vi "Main.vi"() -> ()   [LabVIEW 2022 SP3]
doc: "This Continuous Measurement sample project is based on the Queued Message Handler template.\n\nThe Event Handling Loop generates messages based on user interface actions.\n\nThe Message Handling Loop processes messages generated by the Event Handling Loop, or by other messages. There are also Acquisition and Logging message handling loop subVIs, and a chart updating loop."
uses:
  Settings/Settings.ctl
  Acquisition/Network Configuration.ctl
  Logging/Logging Configuration.ctl
  controls/UI Data.ctl
  controls/UI State.ctl
  Acquisition/Network JSON.ctl
  support/Message Queue/Enqueue Message (Single).vi
  support/Message Queue/Enqueue Message (Array).vi
  <vilib>/Utility/error.llb/Error Cluster From Error Code.vi
  <vilib>/ErrorRing/Error Ring.xnode
  Acquisition/Acquisition.lvlib
  Logging/Logging.lvlib
  Settings/Settings.lvlib
  support/User Event - Stop/User Event - Stop.lvlib
  support/Message Queue/Message Queue.lvlib
  Settings/Settings Dialog.vi
panel:
  in  "Ignite":bool
  in  "Clear Console":bool
  in  "Deactuate 5":bool
  in  "Deactuate 4":bool
  in  "Deactuate 3":bool
  in  "Deactuate 2":bool
  in  "Deactuate 1":bool
  in  "Actuate 5":bool
  in  "Actuate 4":bool
  in  "Actuate 3":bool
  in  "Actuate 2":bool
  out "Pressure Transducers":waveform(dbl)[](graph)
  out "sensors":dbl[](array[numeric])
  out "Ignition State":bool
  out "Switch 5":bool
  out "Switch 4":bool
  out "Switch 3":bool
  out "Switch 2":bool
  out "Switch 1":bool
  out "Temperature":waveform(dbl)[](graph)
  out "Load Cells & Strain Gauges":waveform(dbl)[](graph)
  out "Console":string
  in  "Actuate 1":bool
  in  "Settings":bool
  in  "Restart Remote":bool
  in  "Connect":bool
  in  "Exit":bool
  # "LC 0"
  # "LC 1"
  # "LC 2"
  # "LC 3"
  # "SG 0"
  # "SG 1"
  # "TC 0"
  # "TC 1"
  # "TC 2"
  # "TC 3"
  # "PT 0"
  # "PT 1"
  # "PT 2"
  # "PT 3"
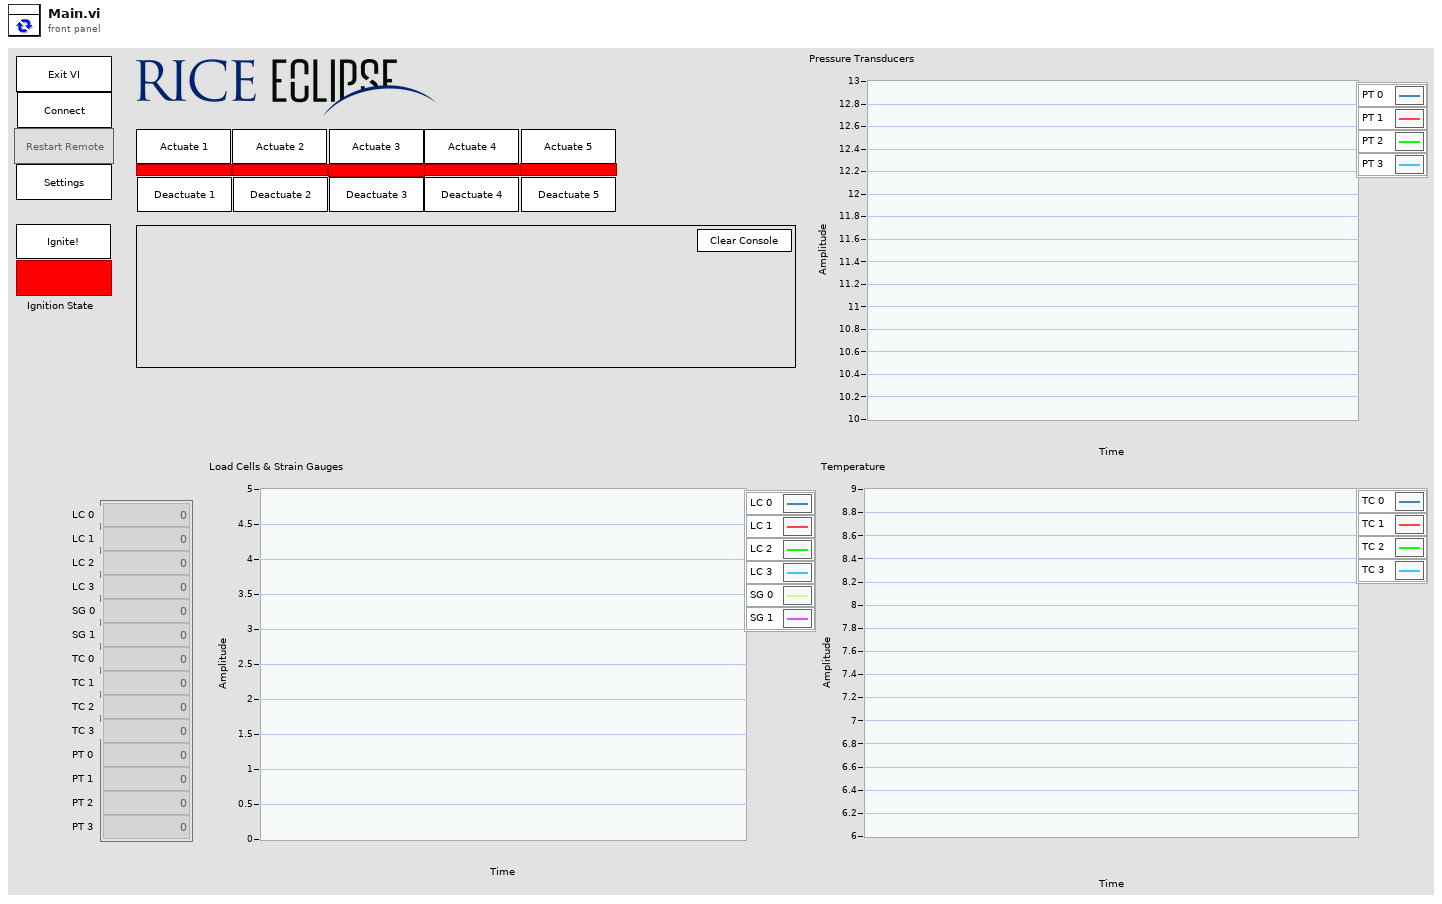
[diagram p1: front panel]
types:
  T1 = typedef "Network JSON.ctl" = cluster{"states":i32[], "timestamp":string, "console":string, "sensors":dbl[]}
  T2 = typedef "UI State.ctl" = enum16{"Idle", "Acquiring and Logging", "Waiting for Exit", "Waiting for Exit (Acq Stopped)", "Waiting for Exit (Log Stopped)", "Waiting for Stop", "Waiting for Stop (Acq Stopped)", "Waiting for Stop (Log Stopped)"}
  T3 = typedef "UI Data.ctl" = cluster{"Start Ref":refnum<vi>, "Stop Ref":refnum<vi>, "Settings Ref":refnum<vi>, "Exit Ref":refnum<vi>, "Console Ref":refnum<vi>, "Data Ref":refnum<vi>}
  T4 = typedef "Settings.lvlib/Settings.ctl" = cluster{"Network Configuration":T5, "Logging Configuration":T6}
  T5 = typedef "Acquisition.lvlib/Network Configuration.ctl" = cluster{"IP Address":string, "Port":dbl, "TCP Network Connection Refnum":refnum<k5>}
  T6 = typedef "Logging.lvlib/Logging Configuration.ctl" = cluster{"Log File Base Path":path, "TDMS File Reference":refnum<k34>}
  T7 = typedef "Message Queue.lvlib/All Message Queues.ctl" = cluster{"UI":refnum<queue>, "Acquisition":refnum<queue>, "Logging":refnum<queue>, "Sending":refnum<queue>}
  T8 = cluster{"command":string, "driver":i32, "value":i32}
  T9 = cluster{"[0]":bool, "[1]":bool, "[2]":bool, "[3]":bool, "[4]":bool, "[5]":bool, "[6]":bool, "[7]":bool, "[8]":bool}
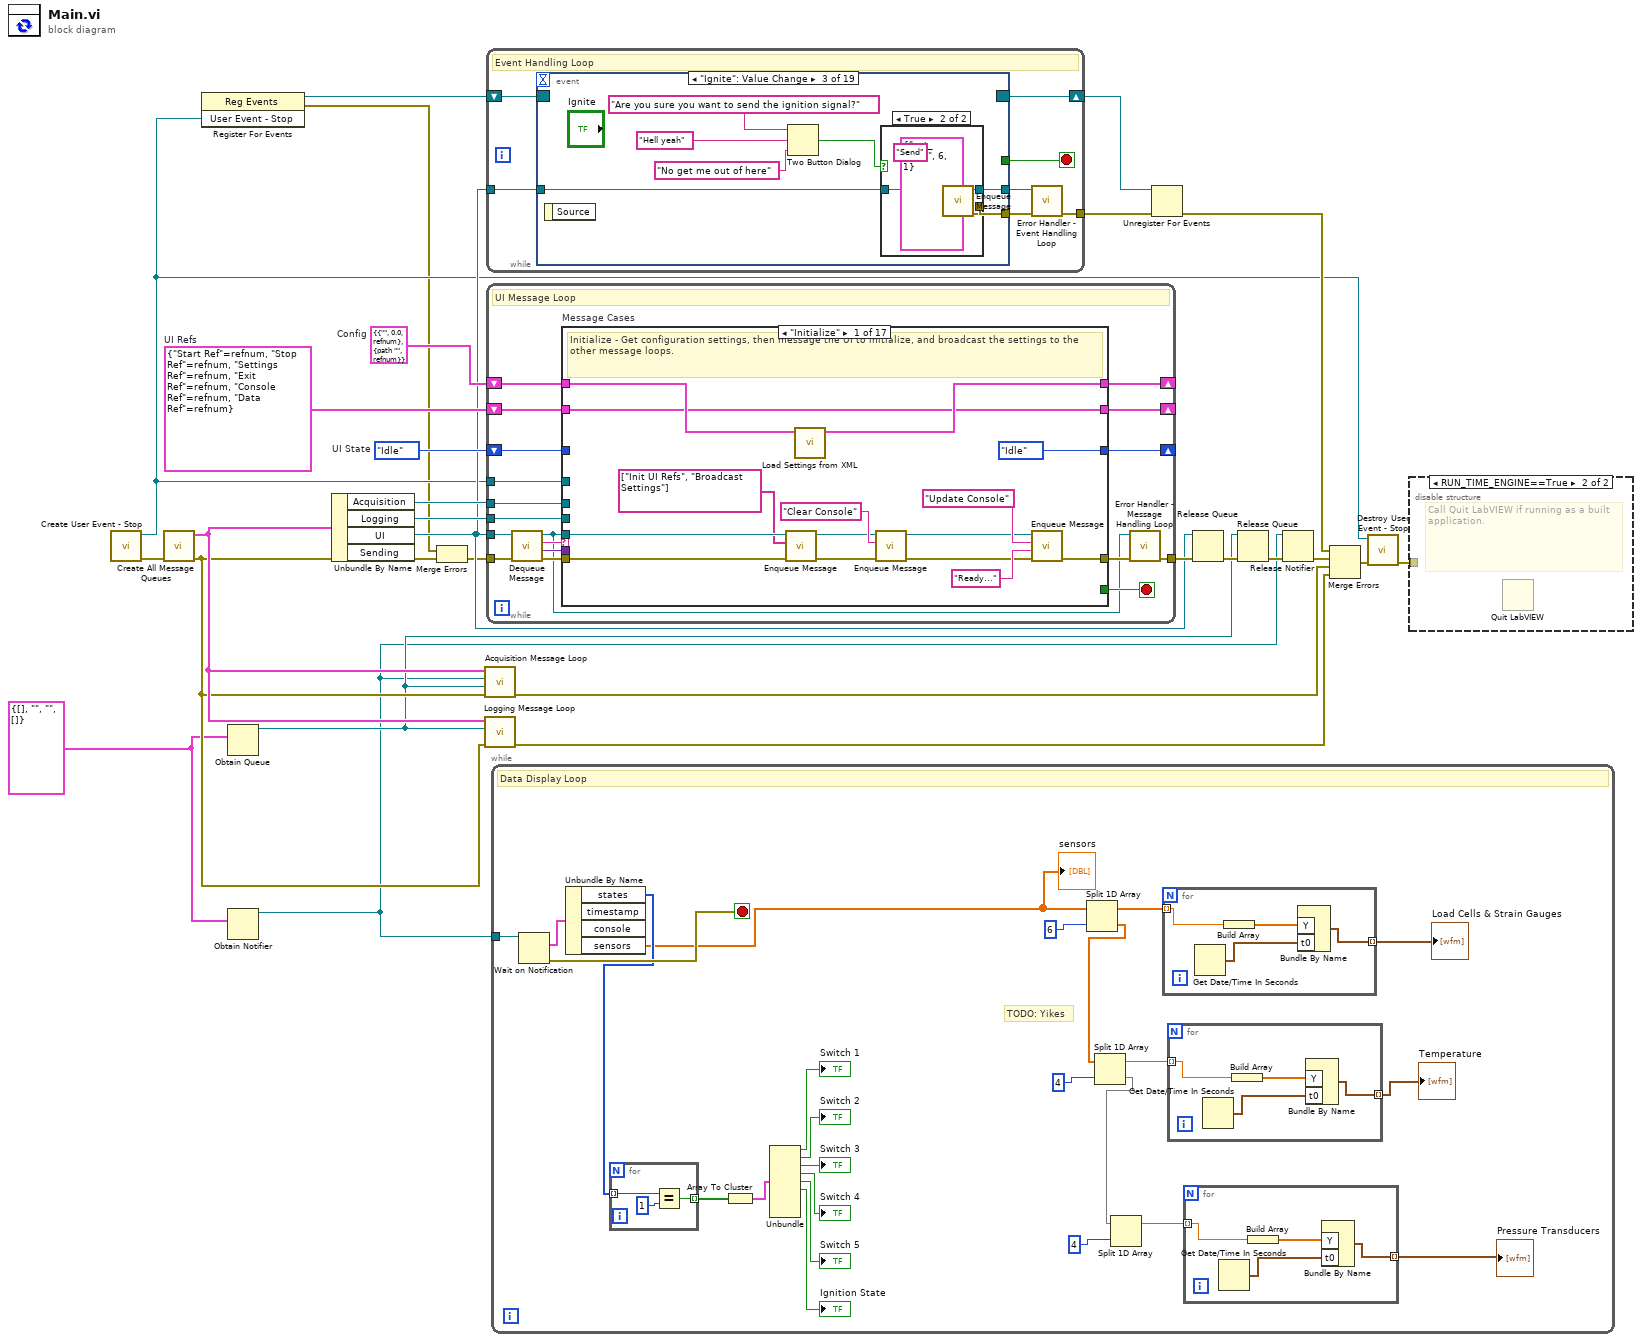
[diagram p0: block diagram]
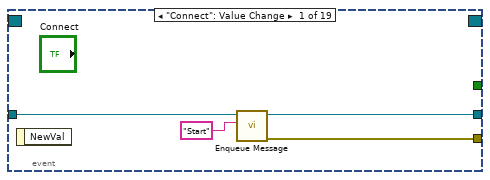
[diagram p3: hidden frame]
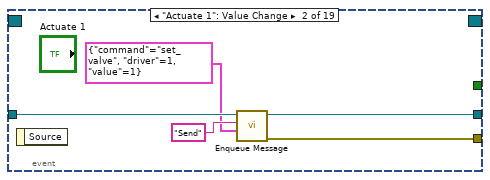
[diagram p4: hidden frame]
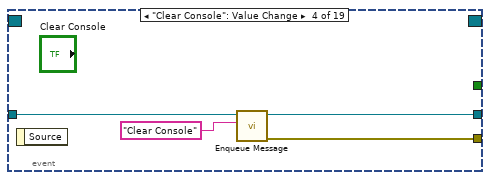
[diagram p6: hidden frame]
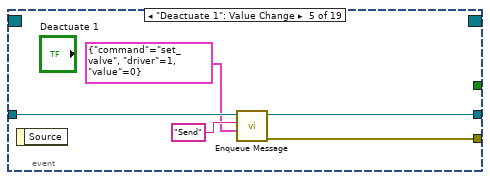
[diagram p7: hidden frame]
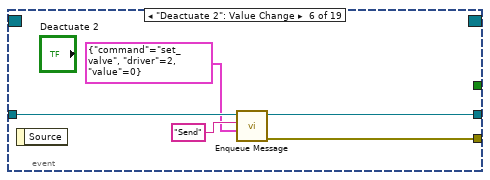
[diagram p8: hidden frame]
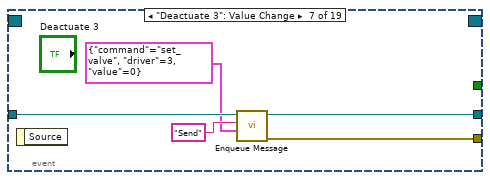
[diagram p9: hidden frame]
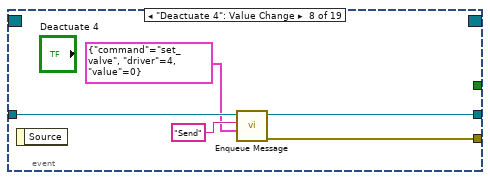
[diagram p10: hidden frame]
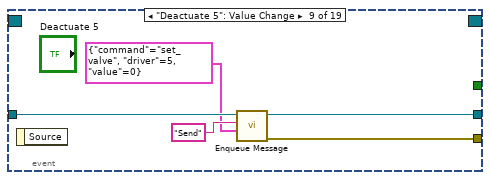
[diagram p11: hidden frame]
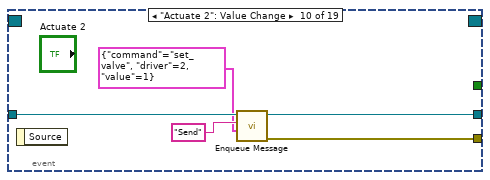
[diagram p12: hidden frame]
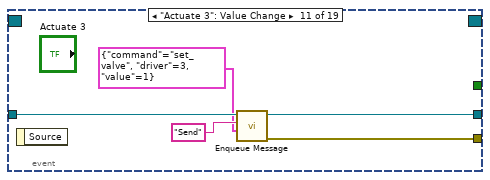
[diagram p13: hidden frame]
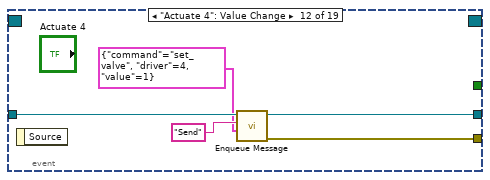
[diagram p14: hidden frame]
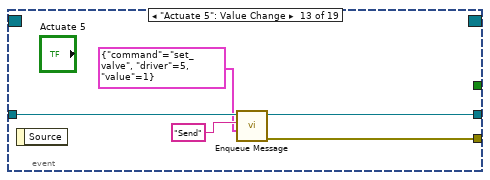
[diagram p15: hidden frame]
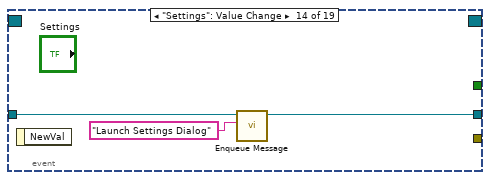
[diagram p16: hidden frame]
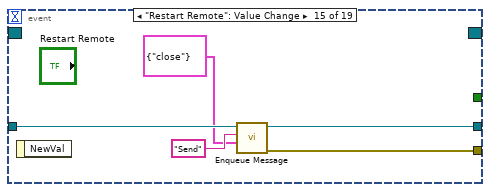
[diagram p17: hidden frame]
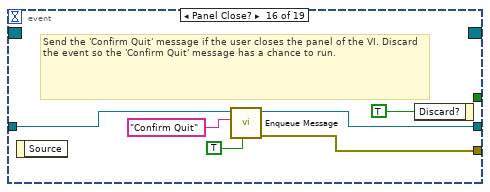
[diagram p18: hidden frame]
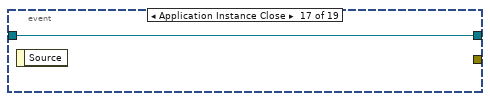
[diagram p19: hidden frame]
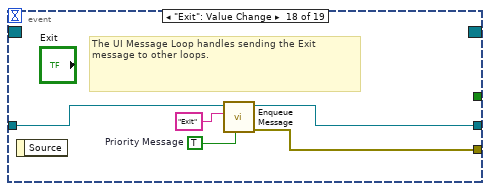
[diagram p20: hidden frame]
diagram:
  w2 = T1 {"states"=[], "timestamp"="", "console"="", "sensors"=[]} ("Network JSON")
  w14 = UI_State."Idle"  # UI State
  w17 = T3 {"Start Ref"=refnum, "Stop Ref"=refnum, "Settings Ref"=refnum, "Exit Ref"=refnum, "Console Ref"=refnum, "Data Ref"=refnum}  # UI Refs
  w20 = T4 {"Network Configuration"={"IP Address"="", "Port"=0.0, "TCP Network Connection Refnum"=refnum}, "Logging Configuration"={"Log File Base Path"=path "", "TDMS File Reference"=refnum}}  # Config
  n1 = call "Create User Event - Stop.vi"() -> ("error out"=w24:errorcluster, "User Event - Stop"=w5:refnum<user-event>)  [unwired: 10 in]
  n2 = call "Create All Message Queues.vi"("error in (no error)"=w24) -> ("error out"=w21:errorcluster, "Message Queues out"=w23:T7)  [unwired: 9 in]
  n3 = register-events(w5) -> (reference out=w6:refnum<event-registration>, error out=w3:errorcluster)  [unwired: 2 in]
  n4 = Obtain Queue(element data type=w2) -> (queue out=w7:refnum<queue>)  [unwired: 4 in, 2 out]
  n5 = Obtain Notifier(notification data type=w2) -> (notifier out=w1:refnum<notifier>)  [unwired: 3 in, 2 out]
  n6 = Unbundle By Name(w23) -> ("Acquisition"=w16:refnum<queue>, "Logging"=w15:refnum<queue>, "UI"=w12:refnum<queue>)  [unwired: 1 out]
  n7 = Merge Errors(w3, w21) -> (w4:errorcluster)
  n8 = call "Acquisition Message Loop.vi"("error in (no error)"=w21, "Data Queue"=w7, "Data Notifier"=w1, "Message Queues"=w23) -> ("error out"=w25:errorcluster)  [unwired: 7 in]
  n9 = call "Logging Message Loop.vi"("error in (no error)"=w21, "Data Queue"=w7, "Message Queues"=w23) -> ("error out"=w22:errorcluster)  [unwired: 8 in]
  n10 = while {
    tunnel: w12 -> [w33]
    tunnel: [w30] -> w26
    shift-right: [w32] -> w18
    shift-left: w6 -> [w34]
    stop <- w31 stop-if-true
    # "Event Handling Loop"
    n11 = event shown="[2] \"Ignite\": Value Change" {
      selector: w34 -> [_ _ _ _ _ _ _ _ _ _ _ _ _ _ _ _ _ _ _]
      dyn-events: [_ _ _ _ _ _ _ _ _ _ _ _ _ _ _ _ _ _ _] -> w32
      timeout: _ -> [_ _ _ _ _ _ _ _ _ _ _ _ _ _ _ _ _ _ _]
      tunnel: [_ _ _ _ _ _ _ _ _ _ _ _ _ _ _ _ _ _ TRUE ("Discard?")] -> w31
      tunnel: w33 -> [w38 w43 w50 w60 w65 w70 w75 w80 w85 w90 w95 w100 w105 w107 w112 w117 w120 w122 w126]
      tunnel: [w36 w41 w49 w58 w63 w68 w73 w78 w83 w88 w93 w98 w103 _ w111 w115 _ w125 _] -> w29
      tunnel: [w35 w40 w48 w57 w62 w67 w72 w77 w82 w87 w92 w97 w102 w106 w110 w116 w120 w121 w126] -> w28
      event "Connect": Value Change {
        n12 = event-data() -> ()  [unwired: 1 in, 1 out]
        n13 = call-poly "Enqueue Message.vi"("Message"="Start", "Message Queue"=w38) -> ("error out"=w36:errorcluster, "dup Message Queue"=w35:refnum<queue>)  [unwired: 8 in]
      }
      event "Actuate 1": Value Change {
        n14 = event-data() -> ()  [unwired: 1 in, 1 out]
        n15 = call-poly "Enqueue Message.vi"("Message Data"=T8 {"command"="set_valve", "driver"=1, "value"=1}, "Message"="Send", "Message Queue"=w43) -> ("error out"=w41:errorcluster, "dup Message Queue"=w40:refnum<queue>)  [unwired: 7 in]
      }
      event "Ignite": Value Change {
        n16 = event-data() -> ()  [unwired: 1 in, 1 out]
        n17 = Two Button Dialog(message="Are you sure you want to send the ignition signal?", 1:"No get me out of here", 2:"Hell yeah") -> (T button?=w44:bool)
        n18 = case shown="True" w44 {
          tunnel: w50 -> [w51 w56]
          tunnel: [_ w54] -> w49
          tunnel: [w51 w53] -> w48
          frame False {
          }
          frame True {
            n19 = call-poly "Enqueue Message.vi"("Message Data"=T8 {"command"="set_valve", "driver"=6, "value"=1}, "Message"="Send", "Message Queue"=w56) -> ("error out"=w54:errorcluster, "dup Message Queue"=w53:refnum<queue>)  [unwired: 7 in]
          }
        }
      }
      event "Clear Console": Value Change {
        n20 = event-data() -> ()  [unwired: 1 in, 1 out]
        n21 = call-poly "Enqueue Message.vi"("Message"="Clear Console", "Message Queue"=w60) -> ("error out"=w58:errorcluster, "dup Message Queue"=w57:refnum<queue>)  [unwired: 8 in]
      }
      event "Deactuate 1": Value Change {
        n22 = event-data() -> ()  [unwired: 1 in, 1 out]
        n23 = call-poly "Enqueue Message.vi"("Message Data"=T8 {"command"="set_valve", "driver"=1, "value"=0}, "Message"="Send", "Message Queue"=w65) -> ("error out"=w63:errorcluster, "dup Message Queue"=w62:refnum<queue>)  [unwired: 7 in]
      }
      event "Deactuate 2": Value Change {
        n24 = event-data() -> ()  [unwired: 1 in, 1 out]
        n25 = call-poly "Enqueue Message.vi"("Message Data"=T8 {"command"="set_valve", "driver"=2, "value"=0}, "Message"="Send", "Message Queue"=w70) -> ("error out"=w68:errorcluster, "dup Message Queue"=w67:refnum<queue>)  [unwired: 7 in]
      }
      event "Deactuate 3": Value Change {
        n26 = event-data() -> ()  [unwired: 1 in, 1 out]
        n27 = call-poly "Enqueue Message.vi"("Message Data"=T8 {"command"="set_valve", "driver"=3, "value"=0}, "Message"="Send", "Message Queue"=w75) -> ("error out"=w73:errorcluster, "dup Message Queue"=w72:refnum<queue>)  [unwired: 7 in]
      }
      event "Deactuate 4": Value Change {
        n28 = event-data() -> ()  [unwired: 1 in, 1 out]
        n29 = call-poly "Enqueue Message.vi"("Message Data"=T8 {"command"="set_valve", "driver"=4, "value"=0}, "Message"="Send", "Message Queue"=w80) -> ("error out"=w78:errorcluster, "dup Message Queue"=w77:refnum<queue>)  [unwired: 7 in]
      }
      event "Deactuate 5": Value Change {
        n30 = event-data() -> ()  [unwired: 1 in, 1 out]
        n31 = call-poly "Enqueue Message.vi"("Message Data"=T8 {"command"="set_valve", "driver"=5, "value"=0}, "Message"="Send", "Message Queue"=w85) -> ("error out"=w83:errorcluster, "dup Message Queue"=w82:refnum<queue>)  [unwired: 7 in]
      }
      event "Actuate 2": Value Change {
        n32 = event-data() -> ()  [unwired: 1 in, 1 out]
        n33 = call-poly "Enqueue Message.vi"("Message Data"=T8 {"command"="set_valve", "driver"=2, "value"=1}, "Message"="Send", "Message Queue"=w90) -> ("error out"=w88:errorcluster, "dup Message Queue"=w87:refnum<queue>)  [unwired: 7 in]
      }
      event "Actuate 3": Value Change {
        n34 = event-data() -> ()  [unwired: 1 in, 1 out]
        n35 = call-poly "Enqueue Message.vi"("Message Data"=T8 {"command"="set_valve", "driver"=3, "value"=1}, "Message"="Send", "Message Queue"=w95) -> ("error out"=w93:errorcluster, "dup Message Queue"=w92:refnum<queue>)  [unwired: 7 in]
      }
      event "Actuate 4": Value Change {
        n36 = event-data() -> ()  [unwired: 1 in, 1 out]
        n37 = call-poly "Enqueue Message.vi"("Message Data"=T8 {"command"="set_valve", "driver"=4, "value"=1}, "Message"="Send", "Message Queue"=w100) -> ("error out"=w98:errorcluster, "dup Message Queue"=w97:refnum<queue>)  [unwired: 7 in]
      }
      event "Actuate 5": Value Change {
        n38 = event-data() -> ()  [unwired: 1 in, 1 out]
        n39 = call-poly "Enqueue Message.vi"("Message Data"=T8 {"command"="set_valve", "driver"=5, "value"=1}, "Message"="Send", "Message Queue"=w105) -> ("error out"=w103:errorcluster, "dup Message Queue"=w102:refnum<queue>)  [unwired: 7 in]
      }
      event "Settings": Value Change {
        n40 = event-data() -> ()  [unwired: 1 in, 1 out]
        n41 = call-poly "Enqueue Message.vi"("Message"="Launch Settings Dialog", "Message Queue"=w107) -> ("dup Message Queue"=w106:refnum<queue>)  [unwired: 8 in, 1 out]
      }
      event "Restart Remote": Value Change {
        n42 = event-data() -> ()  [unwired: 1 in, 1 out]
        n43 = call-poly "Enqueue Message.vi"("Message Data"=cluster{"command":string} {"command"="close"}, "Message"="Send", "Message Queue"=w112) -> ("error out"=w111:errorcluster, "dup Message Queue"=w110:refnum<queue>)  [unwired: 7 in]
      }
      event Panel Close? {
        # "Send the 'Confirm Quit' message if the user closes the panel of the VI. Discard the event so the 'Confirm Quit' message has a chance to run."
        n44 = event-data() -> ()  [unwired: 1 in, 1 out]
        n45 = call-poly "Enqueue Message.vi"("Priority Message? (F)"=TRUE, "Message"="Confirm Quit", "Message Queue"=w117) -> ("error out"=w115:errorcluster, "dup Message Queue"=w116:refnum<queue>)  [unwired: 7 in]
        n46 = event-data("Discard?"=TRUE) -> ()  [unwired: 1 in, 1 out]
      }
      event Application Instance Close {
        n47 = event-data() -> ()  [unwired: 1 in, 1 out]
      }
      event "Exit": Value Change {
        w123 = TRUE  # Priority Message
        # "The UI Message Loop handles sending the Exit message to other loops."
        n48 = event-data() -> ()  [unwired: 1 in, 1 out]
        n49 = call-poly "Enqueue Message.vi"("Priority Message? (F)"=w123, "Message"="Exit", "Message Queue"=w122) -> ("error out"=w125:errorcluster, "dup Message Queue"=w121:refnum<queue>)  [unwired: 7 in]
      }
      event User Event {
        # "The Message Handling Loop processed an \"Exit\" message, which fired this event to stop the Event Handling Loop."
        n50 = event-data() -> ()  [unwired: 1 in, 1 out]
        n51 = local write "Console"("Exit" ("Exit String")) -> ()
      }
    }
    n52 = call "Error Handler - Event Handling Loop.vi"("error in (no error)"=w29, "Message Queue"=w28) -> ("dup error in"=w30:errorcluster)  [unwired: 8 in, 1 out]
  }
  n53 = while {
    tunnel: w12 -> [w140]
    tunnel: w5 -> [w145]
    shift-right: [w139] -> _
    shift-left: w20 -> [w138]
    shift-right: [w136] -> _
    shift-left: w17 -> [w137]
    tunnel: w16 -> [w135]
    tunnel: w15 -> [w134]
    shift-right: [w129] -> _
    shift-left: w14 -> [w130]
    tunnel: w4 -> [w144]
    tunnel: [w133] -> w27
    stop <- w146 stop-if-true
    # "UI Message Loop"
    n54 = call "Dequeue Message.vi"("error in (no error)"=w144, "Message Queue"=w140) -> ("error out"=w143:errorcluster, "Message Data"=w141:variant, "Message"=w142:string, "dup Message Queue"=w131:refnum<queue>)  [unwired: 6 in]
    n55 = case "Message Cases" shown="\"Initialize\"" w142 {
      selector: w142 -> [_ _ _ _ _ _ _ _ _ _ _ _ _ _ _ _ w410]
      tunnel: w131 -> [w155 _ _ w210 _ w235 w260 _ w300 w310 w328 _ _ _ _ w397 _]
      tunnel: w143 -> [w154 w175 w187 w209 w229 w236 w261 w288 w302 w312 w327 w356 w373 w380 w388 w403 _]
      tunnel: [w159 w175 w188 w192 w230 w233 w258 w294 w295 w315 w326 w366 w372 w379 w391 w408 w409] -> w132
      tunnel: [_ _ _ _ _ _ _ _ _ _ _ TRUE _ _ _ _ _] -> w146
      tunnel: w141 -> [_ _ w186 _ _ _ _ _ _ w316 _ w354 _ _ w386 w402 _]
      tunnel: w145 -> [_ _ _ _ _ _ _ _ _ _ _ w367 _ _ _ _ _]
      tunnel: [w160 w174 w183 w208 w228 w239 w264 w292 w299 w320 w331 w365 w371 w378 w382 w405 w413] -> w139
      tunnel: w138 -> [w161 w174 w183 w208 w228 w239 w264 w292 w303 w320 w331 w365 w371 w378 w383 w405 w413]
      tunnel: w137 -> [w156 w173 w182 w205 w227 w238 w263 w286 w297 w319 w330 w364 w370 w375 w390 w407 w412]
      tunnel: [w156 w171 w182 w205 w227 w238 w263 w286 w297 w319 w330 w364 w370 w375 w390 w407 w412] -> w136
      tunnel: w135 -> [_ _ _ w191 w214 _ _ w285 _ _ _ w363 _ _ _ _ _]
      tunnel: w134 -> [_ _ _ w194 w217 _ _ w284 _ _ _ w362 _ _ _ _ _]
      tunnel: w130 -> [_ _ w181 _ w211 w237 w262 w283 w296 w314 w329 _ w369 w377 w389 w406 w411]
      tunnel: [UI_State."Idle" ("UI State") UI_State."Idle" ("UI State") w181 UI_State."Acquiring and Logging" ("UI State") w212 w234 w259 w283 w296 w314 w325 UI_State."Idle" ("UI State") w369 w377 w389 w406 w411] -> w129
      frame "Initialize" {
        # "Initialize - Get configuration settings, then message the UI to initialize, and broadcast the settings to the other message loops."
        n56 = call-poly "Enqueue Message.vi"("error in (no error)"=w154, "Message Array"=string[] ["Init UI Refs", "Broadcast Settings"], "Message Queue"=w155) -> ("error out"=w151:errorcluster, "dup Message Queue"=w148:refnum<queue>)  [unwired: 7 in]
        n57 = call "Load Settings from XML.vi"("Settings in"=w161) -> ("Settings out"=w160:T4)  [unwired: 9 in, 1 out]
        n58 = call-poly "Enqueue Message.vi"("error in (no error)"=w151, "Message"="Clear Console", "Message Queue"=w148) -> ("error out"=w150:errorcluster, "dup Message Queue"=w147:refnum<queue>)  [unwired: 7 in]
        n59 = call-poly "Enqueue Message.vi"("error in (no error)"=w150, "Message Data"="Ready..." ("Ready..."), "Message"="Update Console", "Message Queue"=w147) -> ("error out"=w159:errorcluster)  [unwired: 6 in, 1 out]
      }
      frame "Init UI Refs" {
        # "Enable: Start, Exit, Settings\nDisable: Stop"
        # "Init UI Refs - Store control references for UI controls.  Also enable/disable controls appropriately."
        n60 = control-ref of="Connect"() -> (w165:refnum<vi>)
        n61 = control-ref of="Restart Remote"() -> (w166:refnum<vi>)
        n62 = control-ref of="Settings"() -> (w164:refnum<vi>)
        n63 = control-ref of="Exit"() -> (w163:refnum<vi>)
        n64 = control-ref of="Console"() -> (w172:refnum<vi>)
        n65 = Bundle By Name(cluster=w173, "Start Ref"=w165, "Stop Ref"=w166, "Settings Ref"=w164, "Exit Ref"=w163, "Console Ref"=w172) -> (w171:T3)
        n66 = Build Array(w165, w164, w163) -> (w169:refnum<vi>[])
        n67 = Build Array(w166) -> (w168:refnum<vi>[])
        n68 = call "Set Enable State on Multiple Controls.vi"("Enable?"=TRUE, "Controls"=w169) -> ()  [unwired: 10 in]
        n69 = call "Set Enable State on Multiple Controls.vi"("Enable?"=FALSE, "Controls"=w168) -> ()  [unwired: 10 in]
      }
      frame "Update Console" {
        # "Update Status - Convert the message data to a string to display in the Status indicator."
        n70 = property on="Console" class="Str"() -> ("Text.Text"=w179:string)  [unwired: 2 in, 2 out]
        n71 = Variant To Data(error in=w187, type="", Variant=w186) -> (data=w178:string, error out=w184:errorcluster)
        n72 = Concatenate Strings(w179, "\r\n", w178) -> (→"Console":string)
        n73 = property on="Console" class="Str"("Text.Scroll Position"=1000000) -> ()  [unwired: 2 in, 2 out]
        n74 = Merge Errors(w184) -> (w188:errorcluster)
      }
      frame "Start" {
        # "Message Acquisition and Logging loops to start."
        # "Enable: Stop\nDisable: Start, Exit, Settings"
        # "Start - Enable/Disable buttons appropriately for an acquisition that has started, and update status display."
        n75 = Unbundle By Name(w205) -> ("Stop Ref"=w200:refnum<vi>, "Start Ref"=w199:refnum<vi>, "Exit Ref"=w198:refnum<vi>, "Settings Ref"=w197:refnum<vi>)
        n76 = call-poly "Enqueue Message.vi"("error in (no error)"=w209, "Message Data"="Acquiring and Logging..." ("Acquiring and Logging..."), "Message"="Update Console", "Message Queue"=w210) -> ("error out"=w196:errorcluster)  [unwired: 6 in, 1 out]
        n77 = Build Array(w199, w198, w197) -> (w203:refnum<vi>[])
        n78 = Build Array(w200) -> (w202:refnum<vi>[])
        n79 = call "Set Enable State on Multiple Controls.vi"("Enable?"=TRUE, "Controls"=w202) -> ()  [unwired: 10 in]
        n80 = call "Set Enable State on Multiple Controls.vi"("Enable?"=FALSE, "Controls"=w203) -> ()  [unwired: 10 in]
        n81 = call-poly "Enqueue Message.vi"("error in (no error)"=w196, "Message"="Start", "Message Queue"=w194) -> ("error out"=w193:errorcluster)  [unwired: 7 in, 1 out]
        n82 = call-poly "Enqueue Message.vi"("error in (no error)"=w193, "Message"="Start", "Message Queue"=w191) -> ("error out"=w192:errorcluster)  [unwired: 7 in, 1 out]
      }
      frame "Stop" {
        # "Message Acquisition and Logging loops to stop"
        # "Enable: Start, Exit, Settings\nDisable: Stop"
        # "Stop - Enable/Disable buttons appropriately for an acquisition that has stopped, and update status display."
        n83 = Unbundle By Name(w227) -> ("Stop Ref"=w222:refnum<vi>, "Start Ref"=w221:refnum<vi>, "Exit Ref"=w220:refnum<vi>, "Settings Ref"=w219:refnum<vi>)
        n84 = Build Array(w221, w220, w219) -> (w225:refnum<vi>[])
        n85 = Build Array(w222) -> (w224:refnum<vi>[])
        n86 = call "Set Enable State on Multiple Controls.vi"("Enable?"=FALSE, "Controls"=w224) -> ()  [unwired: 10 in]
        n87 = call "Set Enable State on Multiple Controls.vi"("Enable?"=TRUE, "Controls"=w225) -> ()  [unwired: 10 in]
        n88 = call-poly "Enqueue Message.vi"("error in (no error)"=w229, "Message"="Stop", "Message Queue"=w217) -> ("error out"=w216:errorcluster)  [unwired: 7 in, 1 out]
        n89 = case shown="\"Waiting for Exit\"" w211 {
          selector: w211 -> [w231 _]
          tunnel: [w231 UI_State."Waiting for Stop" ("UI State")] -> w212
          frame "Waiting for Exit" {
          }
          frame Default {
          }
        }
        n90 = call-poly "Enqueue Message.vi"("error in (no error)"=w216, "Message"="Stop", "Message Queue"=w214) -> ("error out"=w215:errorcluster)  [unwired: 7 in, 1 out]
        n91 = Merge Errors(w215) -> (w230:errorcluster)
      }
      frame "Acquisition Stopped" {
        # "Logic for determining what action to take when the acquisition has stopped."
        n92 = case shown="\"Waiting for Exit (Log Stopped)\"" w237 {
          selector: w237 -> [w241 _ _ _ _]
          tunnel: w236 -> [w240 w243 w245 w251 w257]
          tunnel: w235 -> [_ _ _ w249 w254]
          tunnel: [w241 UI_State."Waiting for Exit (Acq Stopped)" ("UI State") UI_State."Waiting for Stop (Acq Stopped)" ("UI State") UI_State."Idle" ("UI State") UI_State."Idle" ("UI State")] -> w234
          tunnel: [w240 w243 w245 w250 w255] -> w233
          frame Default {
          }
          frame "Waiting for Exit", "Waiting for Exit (Acq Stopped)" {
          }
          frame "Waiting for Stop", "Waiting for Stop (Acq Stopped)" {
          }
          frame "Waiting for Exit (Log Stopped)" {
            # "If we are waiting to exit, and the logging has already stopped, then the \"Acquisition Stopped\" message indicates that it is time to exit."
            n93 = call-poly "Enqueue Message.vi"("Priority Message? (F)"=TRUE, "error in (no error)"=w251, "Message"="Exit", "Message Queue"=w249) -> ("error out"=w250:errorcluster)  [unwired: 6 in, 1 out]
          }
          frame "Waiting for Stop (Log Stopped)" {
            # "If we are waiting to stop, and the logging has already stopped, then the \"Acquisition Stopped\" message indicates that it is time to stop."
            n94 = call-poly "Enqueue Message.vi"("error in (no error)"=w257, "Message Data"="Ready..." ("Ready..."), "Message"="Update Status", "Message Queue"=w254) -> ("error out"=w255:errorcluster)  [unwired: 6 in, 1 out]
          }
        }
      }
      frame "Logging Stopped" {
        # "Logic for determining what action to take when the logging has stopped."
        n95 = case shown="\"Waiting for Stop (Acq Stopped)\"" w262 {
          selector: w262 -> [w266 _ _ _ _]
          tunnel: w261 -> [w265 w268 w270 w276 w279]
          tunnel: w260 -> [_ _ _ w274 w278]
          tunnel: [w266 UI_State."Waiting for Exit (Log Stopped)" ("UI State") UI_State."Waiting for Stop (Log Stopped)" ("UI State") UI_State."Idle" ("UI State") UI_State."Idle" ("UI State")] -> w259
          tunnel: [w265 w268 w270 w275 w277] -> w258
          frame Default {
          }
          frame "Waiting for Exit", "Waiting for Exit (Log Stopped)" {
          }
          frame "Waiting for Stop", "Waiting for Stop (Log Stopped)" {
          }
          frame "Waiting for Exit (Acq Stopped)" {
            # "If we are waiting to exit, and the acquisition has already stopped, then the \"Logging Stopped\" message indicates that it is time to exit."
            n96 = call-poly "Enqueue Message.vi"("Priority Message? (F)"=TRUE, "error in (no error)"=w276, "Message"="Exit", "Message Queue"=w274) -> ("error out"=w275:errorcluster)  [unwired: 6 in, 1 out]
          }
          frame "Waiting for Stop (Acq Stopped)" {
            # "If we are waiting to stop, and the acquisition has already stopped, then the \"Logging Stopped\" message indicates that it is time to stop."
            n97 = call-poly "Enqueue Message.vi"("error in (no error)"=w279, "Message Data"="Ready..." ("Ready..."), "Message"="Update Console", "Message Queue"=w278) -> ("error out"=w277:errorcluster)  [unwired: 6 in, 1 out]
          }
        }
      }
      frame "Broadcast settings" {
        w287 = "Update Settings" ("Message")
        # "Broadcast settings - Send the 'Update Settings' message to the Logging and Acquisition message loops."
        n98 = Unbundle By Name(w292) -> ("Network Configuration"=w291:T5, "Logging Configuration"=w290:T6)
        n99 = call-poly "Enqueue Message.vi"("Message Data"=w291, "Message"=w287, "Message Queue"=w285) -> ("error out"=w293:errorcluster)  [unwired: 7 in, 1 out]
        n100 = call-poly "Enqueue Message.vi"("error in (no error)"=w293, "Message Data"=w290, "Message"=w287, "Message Queue"=w284) -> ("error out"=w289:errorcluster)  [unwired: 6 in, 1 out]
        n101 = Merge Errors(w289, w288) -> (w294:errorcluster)
      }
      frame "Launch Settings Dialog" {
        # "Launch Settings Dialog - Launch the Settings Dialog when the user clicks the 'Settings' button."
        n102 = call-by-ref "?"("error in (no error)"=w302, "Settings in"=w303) -> ("error out"=w298:errorcluster, "Cancelled?"=w301:bool, "Settings out"=w299:T4)  [unwired: 8 in, 3 out]
        n103 = case shown="False" w301 {
          tunnel: w300 -> [w307 _]
          tunnel: w298 -> [w306 w308]
          tunnel: [w305 w308] -> w295
          frame False {
            n104 = call-poly "Enqueue Message.vi"("error in (no error)"=w306, "Message"="Broadcast Settings", "Message Queue"=w307) -> ("error out"=w305:errorcluster)  [unwired: 7 in, 1 out]
          }
          frame True {
          }
        }
      }
      frame "Error" {
        # "Error - Display an error dialog. This message is sent by the \"Error Handler\" VIs at the end of other loops in this application."
        n105 = Variant To Data(error in=w312, type=errorcluster {"status"=FALSE, "code"=0, "source"=""} ("error constant"), Variant=w316) -> (data=w313:errorcluster, error out=w317:errorcluster)
        n106 = call <vilib>:"Simple Error Handler.vi"("error in (no error)"=w313) -> ("code out"=w311:i32)  [unwired: 4 in, 4 out]
        n107 = case shown="63" w311 {
          tunnel: w310 -> [_ w323]
          tunnel: [_ w321] -> w309
          frame 0, Default {
          }
          frame 63 {
            n108 = call-poly "Enqueue Message.vi"("Priority Message? (F)"=TRUE, "Message"="Exit", "Message Queue"=w323) -> ("error out"=w321:errorcluster)  [unwired: 7 in, 1 out]
          }
        }
        n109 = Merge Errors(w309, w317) -> (w315:errorcluster)
      }
      frame "Confirm Quit" {
        # "Confirm Quit - Message that can confirm whether or not the user wants to exit the application."
        n110 = case shown="\"Acquiring and Logging\"" w329 {
          tunnel: w328 -> [w337 w341]
          tunnel: w327 -> [w336 w340]
          tunnel: [w335 w339] -> w326
          tunnel: [UI_State."Idle" ("UI State") w338] -> w325
          frame Default {
            # "If 'Confirm Quit' comes in while the system is idle, there is no need for a confirmation message."
            n111 = call-poly "Enqueue Message.vi"("Priority Message? (F)"=TRUE, "error in (no error)"=w336, "Message"="Exit", "Message Queue"=w337) -> ("error out"=w335:errorcluster)  [unwired: 6 in, 1 out]
          }
          frame "Acquiring and Logging" {
            n112 = Two Button Dialog(message="Are you sure you want to quit while the acquisition is running?" ("Confirm Quit Message"), 1:"No" ("No"), 2:"Yes" ("Yes")) -> (T button?=w342:bool)
            n113 = case shown="True" w342 {
              tunnel: w341 -> [_ w351]
              tunnel: w340 -> [w347 w352]
              tunnel: [w347 w350] -> w339
              tunnel: [UI_State."Acquiring and Logging" ("UI State") UI_State."Waiting for Exit" ("UI State")] -> w338
              frame False {
                # "User did not want to quit."
              }
              frame True {
                n114 = call-poly "Enqueue Message.vi"("error in (no error)"=w352, "Message"="Stop", "Message Queue"=w351) -> ("error out"=w350:errorcluster)  [unwired: 7 in, 1 out]
              }
            }
          }
        }
      }
      frame "Exit" {
        w358 = TRUE ("Priority Message? (F)")
        w359 = "Exit" ("Message")
        # "Popup an error dialog if 'Exit' was called as a result of an error."
        # "Stop the VI"
        # "Exit - Send Exit messages to the Acquisition and Logging loops, and fire the user event to stop the Event Handling Loop."
        n115 = Variant To Data(type=errorcluster {"status"=FALSE, "code"=0, "source"=""} ("error constant"), Variant=w354) -> (data=w353:errorcluster)  [unwired: 1 in, 1 out]
        n116 = call <vilib>:"Simple Error Handler.vi"("error in (no error)"=w353) -> ()  [unwired: 4 in, 5 out]
        n117 = call-poly "Enqueue Message.vi"("Priority Message? (F)"=w358, "error in (no error)"=w356, "Message"=w359, "Message Queue"=w363) -> ("error out"=w360:errorcluster)  [unwired: 6 in, 1 out]
        n118 = call-poly "Enqueue Message.vi"("Priority Message? (F)"=w358, "error in (no error)"=w360, "Message"=w359, "Message Queue"=w362) -> ("error out"=w357:errorcluster)  [unwired: 6 in, 1 out]
        n119 = call "Fire User Event - Stop.vi"("error in (no error)"=w357, "User Event - Stop"=w367) -> ("error out"=w366:errorcluster)  [unwired: 9 in]
      }
      frame "---Copy This Frame---" {
        # "Duplicate this frame when creating new messages.  Change this comment in the duplicated frame to describe this message."
        n120 = Merge Errors(w373) -> (w372:errorcluster)
      }
      frame "Clear Console" {
        # "Duplicate this frame when creating new messages.  Change this comment in the duplicated frame to describe this message."
        n121 = Unbundle By Name(w375) -> ("Console Ref"=w374:refnum<vi>)
        n122 = property on="Property Node" class="Str"(reference=w374, "Text.Text"="") -> ()  [unwired: 1 in, 2 out]
        n123 = Merge Errors(w380) -> (w379:errorcluster)
      }
      frame "Update Network Refs" {
        # "Duplicate this frame when creating new messages.  Change this comment in the duplicated frame to describe this message."
        n124 = Variant To Data(error in=w388, type=T5 {"IP Address"="", "Port"=0.0, "TCP Network Connection Refnum"=refnum} ("Network Configuration"), Variant=w386) -> (data=w384:T5, error out=w387:errorcluster)
        n125 = Unbundle By Name(w384) -> ("TCP Network Connection Refnum"=w381:refnum<k5>)
        n126 = Bundle By Name(cluster=w383, "Network Configuration.TCP Network Connection Refnum"=w381) -> (w382:T4)
        n127 = Merge Errors(w387) -> (w391:errorcluster)
      }
      frame "Send" {
        # "Duplicate this frame when creating new messages.  Change this comment in the duplicated frame to describe this message."
        n128 = Unbundle By Name(w405) -> ("Network Configuration.TCP Network Connection Refnum"=w404:refnum<k5>)
        n129 = Variant To Data(error in=w403, type=T8 {"command"="set_valve", "driver"=0, "value"=1}, Variant=w402) -> (data=w393:T8, error out=w395:errorcluster)
        n130 = Flatten To JSON(anything=w393, error in (no error)=w395) -> (JSON string=w392:string, 11:w394:errorcluster)  [unwired: 1 in]
        n131 = TCP Write(connection ID=w404, data in=w392, error in (no error)=w394) -> (error out=w399:errorcluster)  [unwired: 1 in, 2 out]
        n132 = call-poly "Enqueue Message.vi"("error in (no error)"=w399, "Message Data"="Sent command" ("Acquiring and Logging..."), "Message"="Update Console", "Message Queue"=w397) -> ("error out"=w398:errorcluster)  [unwired: 6 in, 1 out]
        n133 = Merge Errors(w398) -> (w408:errorcluster)
      }
      frame Default {
        # "'Default' case only runs if there is a message that isn't defined in any of the other cases.  Output a programming error."
        n134 = xnode "Error Ring"("parameter 0"=w410) -> ("error out"=w409:errorcluster)
      }
    }
    n135 = call "Error Handler - Message Handling Loop.vi"("error in (no error)"=w132, "Message Queue"=w131) -> ("dup error in"=w133:errorcluster)  [unwired: 8 in, 1 out]
  }
  n136 = while "Data Display Loop" {
    tunnel: w1 -> [w444]
    stop <- w443 stop-if-true
    # "TODO: Yikes"
    # "Data Display Loop"
    n137 = Wait on Notification(notifier=w444) -> (notification=w427:T1, error out=w443:errorcluster)  [unwired: 3 in, 2 out]
    n138 = Unbundle By Name(w427) -> ("states"=w426:i32[], "sensors"=w424:dbl[])  [unwired: 2 out]
    "sensors" <- w424
    n139 = for {
      tunnel: w426 -> [w449] mode=indexing
      tunnel: [w451] -> w425 mode=indexing
      n140 = Equal?(x=w449, y=1) -> (x = y?=w451:bool)
    }
    n141 = Array To Cluster(array=w425) -> (cluster=w428:T9)
    n142 = Unbundle(w428) -> ("[0]"=→"Switch 1":bool, "[1]"=→"Switch 2":bool, "[2]"=→"Switch 3":bool, "[3]"=→"Switch 4":bool, "[4]"=→"Switch 5":bool, "[5]"=→"Ignition State":bool)  [unwired: 3 out]
    n143 = Split 1D Array(array=w424, index=6) -> (first subarray=w423:dbl[], second subarray=w439:dbl[])
    n144 = Split 1D Array(array=w439, index=4) -> (first subarray=w440:dbl[], second subarray=w435:dbl[])
    n145 = Split 1D Array(array=w435, index=4) -> (first subarray=w436:dbl[])  [unwired: 1 out]
    n146 = for {
      tunnel: w423 -> [w446] mode=indexing
      tunnel: [w445] -> w422 mode=indexing
      n147 = Get Date/Time In Seconds() -> (seconds since 1Jan1904=w448:timestamp)
      n148 = Build Array(w446) -> (w447:dbl[])
      n149 = Bundle By Name("Y"=w447, "t0"=w448) -> (w445:waveform(dbl))  [unwired: 1 in]
    }
    "Load Cells & Strain Gauges" <- w422
    n150 = for {
      tunnel: w440 -> [w458] mode=indexing
      tunnel: [w457] -> w438 mode=indexing
      n151 = Get Date/Time In Seconds() -> (seconds since 1Jan1904=w459:timestamp)
      n152 = Build Array(w458) -> (w456:dbl[])
      n153 = Bundle By Name("Y"=w456, "t0"=w459) -> (w457:waveform(dbl))  [unwired: 1 in]
    }
    "Temperature" <- w438
    n154 = for {
      tunnel: w436 -> [w454] mode=indexing
      tunnel: [w453] -> w421 mode=indexing
      n155 = Get Date/Time In Seconds() -> (seconds since 1Jan1904=w455:timestamp)
      n156 = Build Array(w454) -> (w452:dbl[])
      n157 = Bundle By Name("Y"=w452, "t0"=w455) -> (w453:waveform(dbl))  [unwired: 1 in]
    }
    "Pressure Transducers" <- w421
  }
  n158 = Unregister For Events(event registration refnum=w18, error in=w26) -> (error out=w19:errorcluster)
  n159 = Release Queue(queue=w12, error in (no error)=w27) -> (error out=w10:errorcluster)  [unwired: 1 in, 2 out]
  n160 = Release Queue(queue=w7, error in (no error)=w10) -> (error out=w9:errorcluster)  [unwired: 1 in, 2 out]
  n161 = Release Notifier(notifier=w1, error in (no error)=w9) -> (error out=w8:errorcluster)  [unwired: 1 in, 2 out]
  n162 = Merge Errors(w19, w8, w25, w22) -> (w13:errorcluster)
  n163 = call "Destroy User Event - Stop.vi"("error in (no error)"=w13, "User Event - Stop"=w5) -> ("error out"=w11:errorcluster)  [unwired: 9 in]
  n164 = disable-structure shown="RUN_TIME_ENGINE==True" {
    disable-tunnel: w11 -> [_ _]
    frame condition #0 (active) {
    }
    frame condition #1 {
      # "Call Quit LabVIEW if running as a built application."
      n165 = Quit LabVIEW() -> ()  [unwired: 1 in]
    }
  }
